vi "Beak Controller.vi"(8 "error in":errorcluster) -> ()   [LabVIEW 2018]
doc: "This VI executes continuously carrying out the current operation and responding to updates or new operations. It will often contain the timing or control code that is difficult to place directly in TeleOp. This VI generally opens all sensors and motors and isolates the rest of the robot code from knowing how the operations are carried out."
uses:
  <vilib>/Rock Robotics/WPI/Framework/Completion Status.ctl
  Beak Setpoints.ctl
  Beak Operations.ctl
  <vilib>/Rock Robotics/WPI/Solenoid/WPI_SolenoidValue.ctl
  <vilib>/Rock Robotics/WPI/Solenoid/WPI_SolenoidDevRef.ctl
  <vilib>/Rock Robotics/WPI/Solenoid/WPI_SolenoidChannel.ctl
  <vilib>/Rock Robotics/WPI/Counter/WPI_CounterDevRef.ctl
  <vilib>/Rock Robotics/SystemInterfaces/Counter/FPGA_CounterCtrSystemIndex.ctl
  <vilib>/Rock Robotics/WPI/Solenoid/WPI_SolenoidSetEnum.vi
  Beak Published Globals.vi
  Wrist/Implementation/Wrist Published Globals.vi
panel:
  in  "Wrist Block Angle":dbl=60.0
  in  "Sensor Distance mm":dbl=60.0
  out "Waveform Chart":dbl(graph)
  out "Distance mm":dbl
  in  "Extend Polarity":T1=enum."Reverse"
  in  "Open Polarity":T1=enum."Reverse"
  in  "Interactive Values":T2
  out "Current\nCmd":string
  in  "Buttons":cluster{"Execute Cmd":bool, "Abort Cmd":bool}
  out "Command Timing":cluster{"Start Time (ms)":u32, "Iterations":i32}
  out "Status":T4
  # "Interactive Command: You may fill in the settings for a command\nand schedule it with the Execute button. You can observe and abort\nany command while fine tuning the code for the controller."
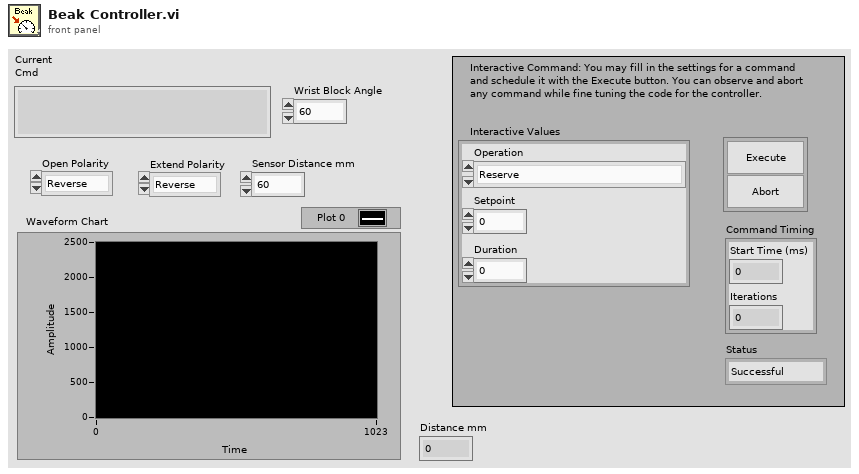
[diagram p1: front panel]
types:
  T1 = typedef "WPI_SolenoidValue.ctl" = enum16{"Off", "On", "Forward", "Reverse"}
  T2 = typedef "Beak Setpoints.ctl" = cluster{"Operation":T3, "Setpoint":dbl, "Duration":dbl}
  T3 = typedef "Beak Operations.ctl" = enum16{"Reserve", "Read Current", "Immediate", "Open", "Close", "Extend", "Retract"}
  T4 = typedef "Completion Status.ctl" = enum16{"Successful", "Aborted", "Incomplete"}
  T5 = typedef "WPI_SolenoidDevRef.ctl" = cluster{"DevStatus":errorcluster, "Pneumatics Control Module":u8, "Forward Solenoid Channel":T6, "Reverse Solenoid Channel":T6}
  T6 = typedef "WPI_SolenoidChannel.ctl" = enum8{"Solenoid 0", "Solenoid 1", "Solenoid 2", "Solenoid 3", "Solenoid 4", "Solenoid 5", "Solenoid 6", "Solenoid 7", "Invalid"}
  T7 = typedef "WPI_CounterDevRef.ctl" = cluster{"DevStatus":errorcluster, "CntIndex":T8}
  T8 = typedef "FPGA_CounterCtrSystemIndex.ctl" = enum8{"Ctr 0", "Ctr 1", "Ctr 2", "Ctr 3", "Ctr 4", "Ctr 5", "Ctr 6", "Ctr 7", "Invalid"}
  T9 = cluster{"Beak":T5, "BeakExtension":T5, "Hatch Sensor":T7}
  T10 = typedef "Command Status Info.ctl" = cluster{"Name":string, "Status":T4, "notifier out":T11}
  T11 = typedef "Completion Notifier.ctl" = refnum<notifier>
  T12 = cluster{"Current Command":T2, "Command Timing":cluster{"Start Time (ms)":u32, "Iterations":i32}, "Command Arguments":cluster{"Command Info":T10, "Description":string, "Default Command":T2, "queue out":refnum<queue>, "Subsystem Name":string}}
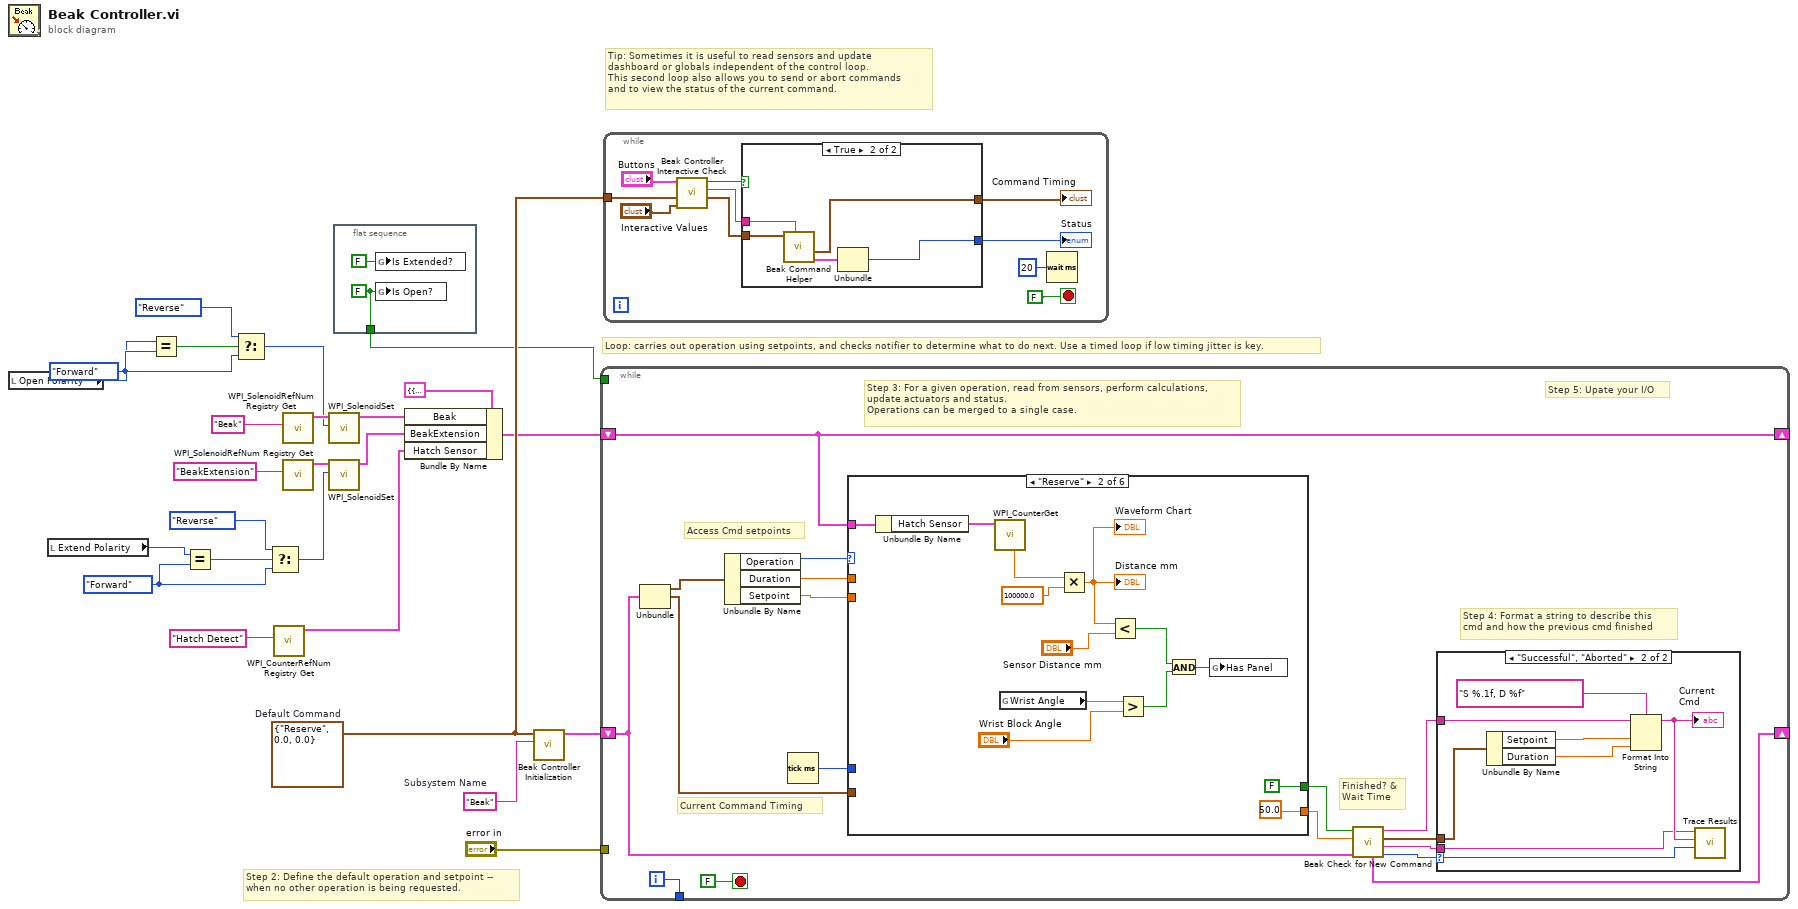
[diagram p0: block diagram]
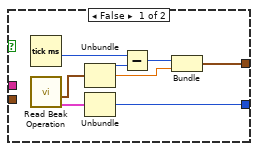
[diagram p2: hidden frame]
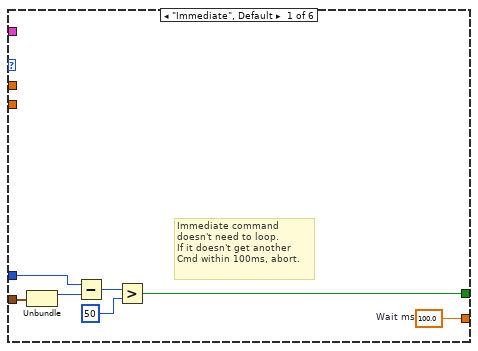
[diagram p4: hidden frame]
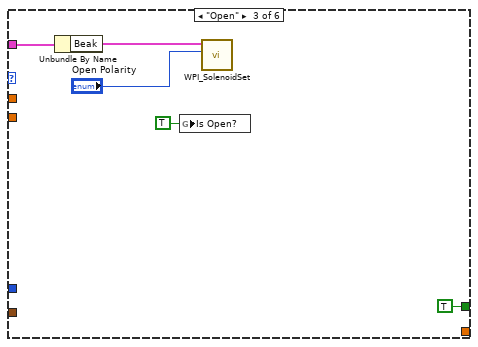
[diagram p5: hidden frame]
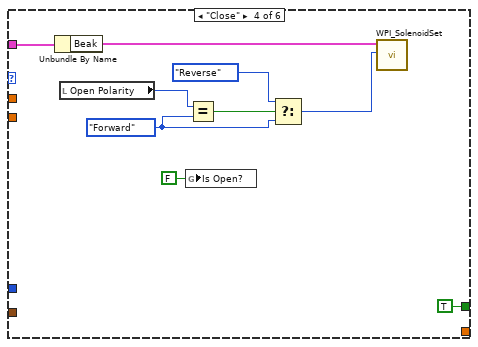
[diagram p6: hidden frame]
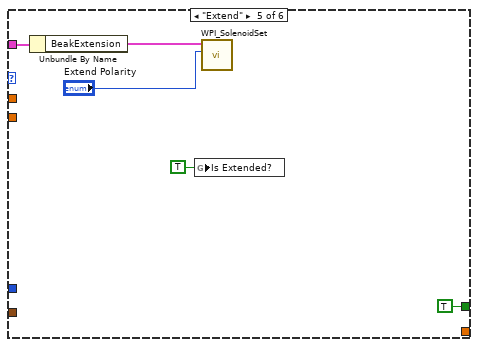
[diagram p7: hidden frame]
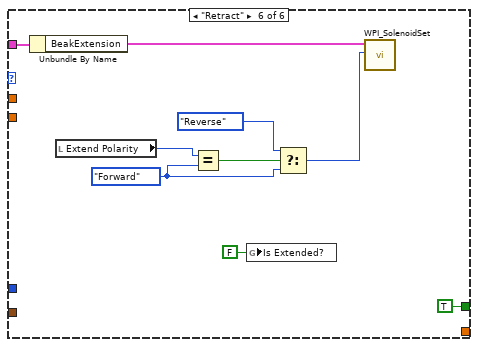
[diagram p8: hidden frame]
diagram:
  w3 = WPI_SolenoidValue."Forward" ("y")
  w13 = WPI_SolenoidValue."Forward" ("y")
  w22 = T2 {"Operation"=enum."Reserve", "Setpoint"=0.0, "Duration"=0.0}  # Default Command
  w23 = "Beak"  # Subsystem Name
  # "Tip: Sometimes it is useful to read sensors and update\ndashboard or globals independent of the control loop.\nThis second loop also allows you to send or abort commands\nand to view the status of the current command."
  # "Step 2: Define the default operation and setpoint --\nwhen no other operation is being requested."
  # "Loop: carries out operation using setpoints, and checks notifier to determine what to do next. Use a timed loop if low timing jitter is key."
  n1 = local read "Open Polarity"() -> (w1:T1)
  n2 = local read "Extend Polarity"() -> (w10:T1)
  n3 = Equal?(x=w1, y=w3) -> (x = y?=w5:bool)
  n4 = Equal?(x=w10, y=w13) -> (x = y?=w11:bool)
  n5 = Select(t=WPI_SolenoidValue."Reverse" ("y"), s=w5, f=w3) -> (s? t:f=w2:T1)
  n6 = Select(t=WPI_SolenoidValue."Reverse" ("y"), s=w11, f=w13) -> (s? t:f=w9:T1)
  n7 = call <vilib>:"WPI_CounterRefNum Registry Get.vi"("refnum name"="Hatch Detect") -> ("CounterDevRef"=w7:T7)  [unwired: 9 in, 1 out]
  n8 = call <vilib>:"WPI_SolenoidRefNum Registry Get.vi"("refnum name"="Beak") -> ("SolenoidDevRef"=w17:T5)  [unwired: 9 in, 1 out]
  n9 = call <vilib>:"WPI_SolenoidRefNum Registry Get.vi"("refnum name"="BeakExtension") -> ("SolenoidDevRef"=w15:T5)  [unwired: 9 in, 1 out]
  n10 = call-poly <vilib>:"WPI_SolenoidSet.vi"("Value"=w2, "SolenoidDevRef"=w17) -> ("SolenoidDevRef"=w16:T5)  [unwired: 8 in, 1 out]
  n11 = call-poly <vilib>:"WPI_SolenoidSet.vi"("Value"=w9, "SolenoidDevRef"=w15) -> ("SolenoidDevRef"=w14:T5)  [unwired: 8 in, 1 out]
  n12 = flat-sequence {
    tunnel: [w26] -> w6
    frame #0 {
      w26 = FALSE ("Is Open?")
      n13 = global write "Beak Published Globals.vi" "Is Extended?"(FALSE ("Is Extended?")) -> ()
      n14 = global write "Beak Published Globals.vi" "Is Open?"(w26) -> ()
    }
  }
  n15 = Bundle By Name(cluster=T9 {"Beak"={"DevStatus"={"status"=FALSE, "code"=0, "source"=""}, "Pneumatics Control Module"=0, "Forward Solenoid Channel"=enum."Invalid", "Reverse Solenoid Channel"=enum."Invalid"}, "BeakExtension"={"DevStatus"={"status"=FALSE, "code"=0, "source"=""}, "Pneumatics Control Module"=0, "Forward Solenoid Channel"=enum."Invalid", "Reverse Solenoid Channel"=enum."Invalid"}, "Hatch Sensor"={"DevStatus"={"status"=FALSE, "code"=0, "source"=""}, "CntIndex"=enum."Ctr 0"}}, "Beak"=w16, "BeakExtension"=w14, "Hatch Sensor"=w7) -> (w18:T9)
  n16 = call "Beak Controller Initialization.vi"("Subsystem Name"=w23, "Default Command"=w22) -> ("Current Command"=w24:T12)  [unwired: 9 in]
  n17 = while {
    shift-right: [w36] -> _
    shift-left: w24 -> [w29]
    tunnel: [w43] -> _
    tunnel: "error in" -> [_]
    shift-right: [w28] -> _
    shift-left: w18 -> [w28]
    tunnel: w6 -> [_]
    i -> [w43]
    stop <- FALSE stop-if-true
    # "Step 5: Upate your I/O"
    # "Step 4: Format a string to describe this\ncmd and how the previous cmd finished"
    # "Current Command Timing"
    # "Access Cmd setpoints"
    # "Finished? &\nWait Time"
    # "Step 3: For a given operation, read from sensors, perform calculations,\nupdate actuators and status.\nOperations can be merged to a single case."
    n18 = Unbundle(w29) -> ("Current Command"=w42:T2, "Command Timing"=w38:cluster{"Start Time (ms)":u32, "Iterations":i32})  [unwired: 1 out]
    n19 = Unbundle By Name(w42) -> ("Operation"=w41:T3, "Duration"=w40:dbl, "Setpoint"=w37:dbl)
    n20 = Tick Count (ms)() -> (millisecond timer value=w39:u32)
    n21 = case shown="\"Reserve\"" w41 {
      tunnel: [w59 50.0 _ _ _ _] -> w34
      tunnel: [w53 FALSE ("ignore previous (F)") TRUE ("ignore previous (F)") TRUE ("ignore previous (F)") TRUE ("ignore previous (F)") TRUE ("ignore previous (F)")] -> w35
      tunnel: w38 -> [w55 _ _ _ _ _]
      tunnel: w40 -> [_ _ _ _ _ _]
      tunnel: w39 -> [w54 _ _ _ _ _]
      tunnel: w37 -> [_ _ _ _ _ _]
      tunnel: w28 -> [_ w70 w77 w86 w91 w100]
      frame "Immediate", Default {
        w59 = 100.0  # Wait ms
        # "Immediate command\ndoesn't need to loop.\nIf it doesn't get another\nCmd within 100ms, abort."
        n22 = Unbundle(w55) -> ("Start Time (ms)"=w58:u32)  [unwired: 1 out]
        n23 = Subtract(x=w54, y=w58) -> (x-y=w57:u32)
        n24 = Greater?(x=w57, y=u8 50 ("Left Motor")) -> (0:w53:bool)
      }
      frame "Reserve" {
        n25 = Unbundle By Name(w70) -> ("Hatch Sensor"=w68:T7)
        n26 = call <vilib>:"WPI_CounterGet.vi"("CounterDevRef in"=w68) -> ("Period (sec)"=w67:dbl)  [unwired: 5 in, 5 out]
        n27 = global read "Wrist Published Globals.vi" "Wrist Angle"() -> (w64:dbl)
        n28 = Multiply(x=w67, y=100000.0) -> (x*y=w66:dbl)
        "Distance mm" <- w66
        "Waveform Chart" <- w66
        n29 = Less?(x=w66, y="Sensor Distance mm") -> (x < y?=w62:bool)
        n30 = Greater?(x=w64, y="Wrist Block Angle") -> (0:w61:bool)
        n31 = And(x=w62, y=w61) -> (x .and. y?=w60:bool)
        n32 = global write "Beak Published Globals.vi" "Has Panel"(w60) -> ()
      }
      frame "Open" {
        n33 = Unbundle By Name(w77) -> ("Beak"=w76:T5)
        n34 = global write "Beak Published Globals.vi" "Is Open?"(TRUE ("Is Open?")) -> ()
        n35 = call-poly <vilib>:"WPI_SolenoidSet.vi"("Value"="Open Polarity", "SolenoidDevRef"=w76) -> ()  [unwired: 8 in, 2 out]
      }
      frame "Close" {
        w82 = WPI_SolenoidValue."Forward" ("y")
        n36 = Unbundle By Name(w86) -> ("Beak"=w85:T5)
        n37 = local read "Open Polarity"() -> (w80:T1)
        n38 = global write "Beak Published Globals.vi" "Is Open?"(FALSE ("Is Open?")) -> ()
        n39 = Equal?(x=w80, y=w82) -> (x = y?=w84:bool)
        n40 = Select(t=WPI_SolenoidValue."Reverse" ("y"), s=w84, f=w82) -> (s? t:f=w81:T1)
        n41 = call-poly <vilib>:"WPI_SolenoidSet.vi"("Value"=w81, "SolenoidDevRef"=w85) -> ()  [unwired: 8 in, 2 out]
      }
      frame "Extend" {
        n42 = Unbundle By Name(w91) -> ("BeakExtension"=w90:T5)
        n43 = global write "Beak Published Globals.vi" "Is Extended?"(TRUE ("Is Extended?")) -> ()
        n44 = call-poly <vilib>:"WPI_SolenoidSet.vi"("Value"="Extend Polarity", "SolenoidDevRef"=w90) -> ()  [unwired: 8 in, 2 out]
      }
      frame "Retract" {
        w95 = WPI_SolenoidValue."Forward" ("y")
        n45 = Unbundle By Name(w100) -> ("BeakExtension"=w99:T5)
        n46 = local read "Extend Polarity"() -> (w98:T1)
        n47 = Equal?(x=w98, y=w95) -> (x = y?=w97:bool)
        n48 = global write "Beak Published Globals.vi" "Is Extended?"(FALSE ("Is Extended?")) -> ()
        n49 = Select(t=WPI_SolenoidValue."Reverse" ("y"), s=w97, f=w95) -> (s? t:f=w94:T1)
        n50 = call-poly <vilib>:"WPI_SolenoidSet.vi"("Value"=w94, "SolenoidDevRef"=w99) -> ()  [unwired: 8 in, 2 out]
      }
    }
    n51 = call "Beak Check for New Command.vi"("Current Command"=w29, "Wait time (ms)"=w34, "Finished?"=w35) -> ("Completion"=w30:T4, "Subsystem Name"=w31:string, "Current Command"=w32:T2, "Initial Trace String"=w33:string, "NextCommand"=w36:T12)  [unwired: 4 in]
    n52 = case shown="\"Successful\", \"Aborted\"" w30 {
      selector: w30 -> [_ w52]
      tunnel: w33 -> [_ w48]
      tunnel: w32 -> [_ w49]
      tunnel: w31 -> [_ w45]
      frame "Incomplete", Default {
        # "Continuing current command"
      }
      frame "Successful", "Aborted" {
        # "Report and setup for next command"
        n53 = Unbundle By Name(w49) -> ("Setpoint"=w51:dbl, "Duration"=w46:dbl)
        n54 = Format Into String(format string="S %.1f, D %f", initial string=w48, w51, w46) -> (resulting string=w47:string)  [unwired: 1 in, 1 out]
        "Current\nCmd" <- w47
        n55 = call <vilib>:"Trace Results.vi"("Status of previous command"=w52, "Description"=w47, "Subsystem"=w45) -> ()  [unwired: 9 in]
      }
    }
  }
  n56 = while {
    tunnel: w22 -> [w107]
    stop <- FALSE stop-if-true
    n57 = call "Beak Controller Interactive Check.vi"("Interactive Command in"="Interactive Values", "Default Command"=w107, "Buttons"="Buttons") -> ("Interactive Command out"=w104:T2, "Trace String"=w105:string, "Schedule"=w106:bool)  [unwired: 6 in]
    n58 = case shown="True" w106 {
      tunnel: [w118 w123] -> w103
      tunnel: w104 -> [_ w121]
      tunnel: [w114 w119] -> w102
      tunnel: w105 -> [_ w122]
      frame False {
        n59 = Tick Count (ms)() -> (millisecond timer value=w113:u32)
        n60 = call "Read Beak Operation.vi"() -> ("Command Info"=w111:T10, "SubSystem Data"=w112:T2)  [unwired: 9 in, 1 out]
        n61 = Unbundle(w112) -> ("Operation"=w117:T3, "Setpoint"=w115:dbl)  [unwired: 1 out]
        n62 = Unbundle(w111) -> ("Status"=w118:T4)  [unwired: 2 out]
        n63 = Subtract(x=w113, y=w117) -> (x-y=w116:u32)
        n64 = Bundle(w116, "Setpoint"=w115) -> (w114:cluster{u32, "Setpoint":dbl})  [unwired: 1 in]
      }
      frame True {
        n65 = call "Beak Command Helper.vi"("Description"=w122, "SubSystem Data"=w121) -> ("Command Info Out"=w120:T10, "Command Timing"=w119:cluster{"Start Time (ms)":u32, "Iterations":i32})  [unwired: 7 in, 1 out]
        n66 = Unbundle(w120) -> ("Status"=w123:T4)  [unwired: 2 out]
      }
    }
    "Status" <- w103
    "Command Timing" <- w102
    n67 = Wait (ms)(milliseconds to wait=u32 20) -> ()  [unwired: 1 out]
  }
